vi "BeadCoolerFixedZ(SubVI).vi"(0 "hp coeff band":i32[](array[numeric])=[-850883994, 1909449570, 958518847, -975456236, 2033039520, 1020559395], 1 "lp coeff band":i32[](array[numeric])=[-955995012, 2025731616, 1001305, -1023351008, 2092954700, 1034533], 2 "ig":fxp<+/-,24,6>, 3 "dg":fxp<+/-,24,12>, 5 "pg":fxp<+/-,24,12>, 6 "dg band":fxp<+/-,24,12>, 10 "AI0":i16, 12 "Dc Pos":i16, 13 "Upper lim":fxp<+/-,16,16>, 16 "lp coeff":i32[](array[numeric])=[1008310688, 32715568], 17 "Lower lim":fxp<+/-,16,16>, 18 "final filter coeff":i32[](array[numeric])=[-955995012, 2025731616, 1001305, -1023351008, 2092954700, 1034533], 23 "hp coeff":i32[](array[numeric])=[946630756, 1010186290]) -> (25 "Output":fxp<+/-,16,16>)   [LabVIEW 2016]
uses:
  <vilib>/rvi/FXPMathLib/basic elements/FxpIntAccumulator/subVIs/nifxpmath_IntAccumulator_SimConfig.ctl
  <vilib>/rvi/FXPMathLib/basic elements/FxpIntAccumulator/simVIs/DllFxpIntAccumulator_sub.vi
  <vilib>/rvi/FXPMathLib/FxpInterpret/XNode/nifxpmath_Interpret.xnode
  <vilib>/rvi/FXPMathLib/basic elements/FxpIntAccumulator/XNode/nifxpmath_IntAccumulator.xnode
  <vilib>/rvi/Analysis/measure/butterworth/XNode/niFpgaButterworthFilter.xnode
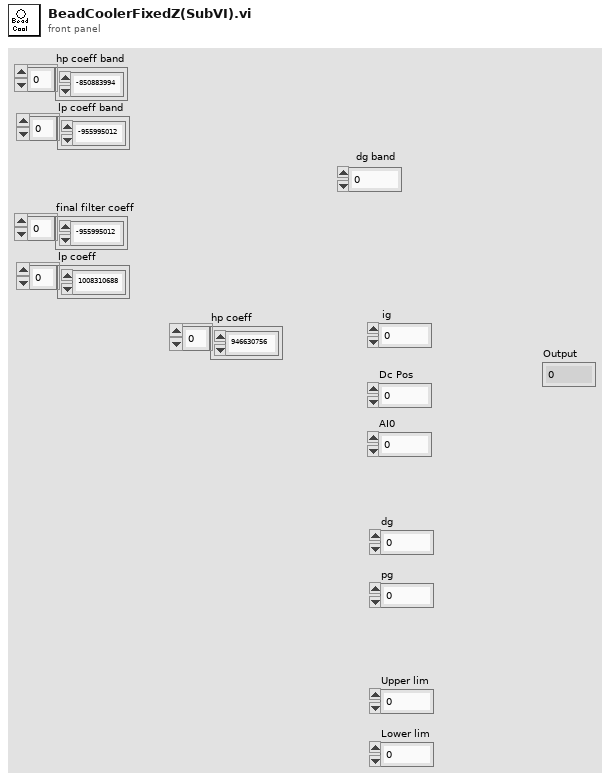
[diagram p1: front panel]
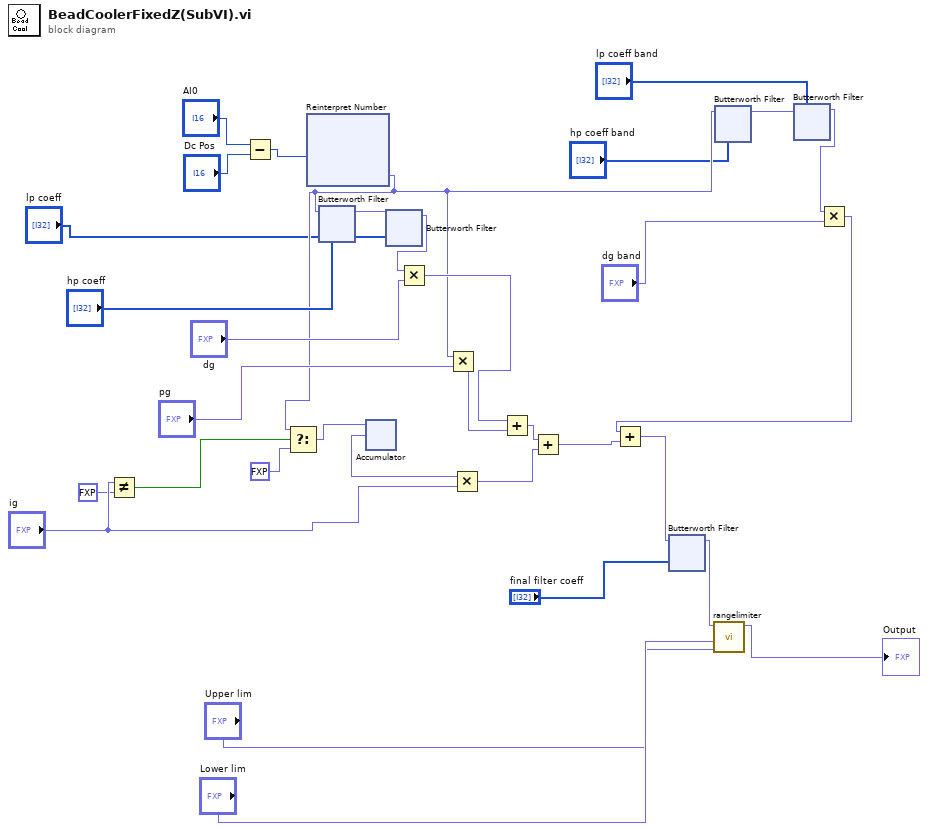
[diagram p0: block diagram]
diagram:
  n1 = Not Equal?(x="ig", y=fxp<+/-,24,6> 0.0) -> (x != y?=w15:bool)
  n2 = Subtract(x="AI0", y="Dc Pos") -> (x-y=w27:i16)
  n3 = xnode "Reinterpret Number"("x"=w27) -> ("y"=w12:fxp<+/-,16,16>)
  n4 = Select(t=w12, s=w15, f=fxp<+/-,16,16> 0.0) -> (s? t:f=w17:fxp<+/-,16,16>)
  n5 = xnode "Butterworth Filter"("input data"=w12, "scaled coefficients"="hp coeff") -> ("output data"=w20:fxp<+/-,16,16>)  [unwired: 1 in]
  n6 = xnode "Accumulator"("x"=w17) -> ("s"=w22:fxp<+/-,32,32>)  [unwired: 4 in, 1 out]
  n7 = xnode "Butterworth Filter"("input data"=w20, "scaled coefficients"="lp coeff") -> ("output data"=w19:fxp<+/-,16,16>)  [unwired: 1 in]
  n8 = Multiply(x=w19, y="dg") -> (x*y=w18:fxp<+/-,18,16>)
  n9 = Multiply(x=w12, y="pg") -> (x*y=w33:fxp<+/-,18,16>)
  n10 = Multiply(x=w22, y="ig") -> (x*y=w23:fxp<+/-,18,16>)
  n11 = Add(x=w18, y=w33) -> (x+y=w24:fxp<+/-,18,16>)
  n12 = Add(x=w24, y=w23) -> (x+y=w7:fxp<+/-,16,16>)
  n13 = xnode "Butterworth Filter"("input data"=w12, "scaled coefficients"="hp coeff band") -> ("output data"=w11:fxp<+/-,16,16>)  [unwired: 1 in]
  n14 = xnode "Butterworth Filter"("input data"=w11, "scaled coefficients"="lp coeff band") -> ("output data"=w10:fxp<+/-,16,16>)  [unwired: 1 in]
  n15 = Multiply(x=w10, y="dg band") -> (x*y=w8:fxp<+/-,18,16>)
  n16 = Add(x=w8, y=w7) -> (x+y=w4:fxp<+/-,16,16>)
  n17 = xnode "Butterworth Filter"("input data"=w4, "scaled coefficients"="final filter coeff") -> ("output data"=w3:fxp<+/-,16,16>)  [unwired: 1 in]
  n18 = call "rangelimiter.vi"("Upper lim"="Upper lim", "Lower lim"="Lower lim", "Input"=w3) -> ("Output"=→"Output":fxp<+/-,16,16>)  [unwired: 8 in]
